vi "Autonomous Independent.vi"() -> ()   [LabVIEW 2015]
doc: "This VI is called when autonomous begins, and will automatically be terminated when autonomous ends. You can carry out timed or sensor driven robot movement independently without needing to return to the caller."
uses:
  <vilib>/Rock Robotics/WPI/Utilities/WPI_GetSetVariantRefNum.vi
  <vilib>/Rock Robotics/Network Tables/NT Read String.vi
  <vilib>/Rock Robotics/Network Tables/NT Write Numeric Array.vi
  <vilib>/Rock Robotics/WPI/RobotDrive/WPI_RobotDriveArcadeDrive_Standard(NoSaturation).vi
  Robot Global Data.vi
panel:
  out "Current Movement, for debugging":T1 {"Y Joystick Value" scale=1.0..-1.0; "X Joystick Value" scale=-1.0..1.0}
  in  "Array of robot movements":T2(array[cluster])=[{"X Joystick Value"=0.39393939393939403, "Y Joystick Value"=0.0, "Delay (sec)"=1.0, "Movement Name"="turn"}, {"X Joystick Value"=-0.3737373737373737, "Y Joystick Value"=0.0, "Delay (sec)"=1.0, "Movement Name"="turn back"}] {"Y Joystick Value" scale=1.0..-1.0; "X Joystick Value" scale=-1.0..1.0}
  # "Be sure to right-click and choose Data Operations>>Make Current Value default if you want to save the array values with the VI"
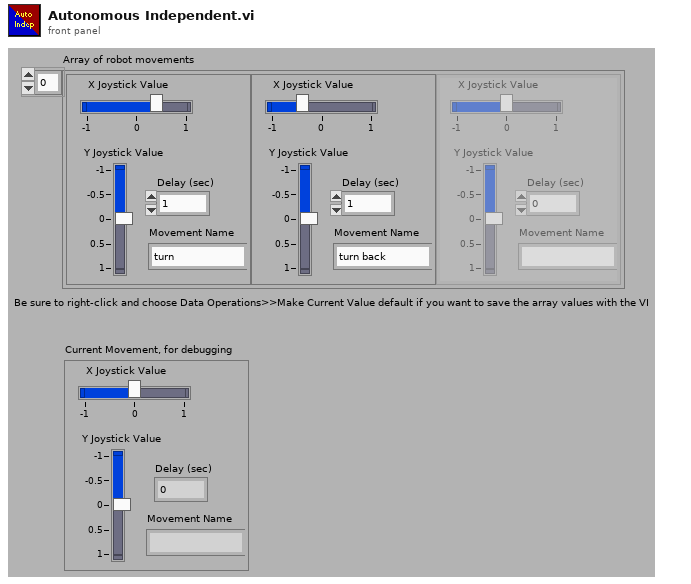
[diagram p1: front panel]
types:
  T1 = cluster{"X Joystick Value":dbl, "Y Joystick Value":dbl, "Delay (sec)":dbl, "Movement Name":string}
  T2 = cluster{"X Joystick Value":dbl, "Y Joystick Value":dbl, "Delay (sec)":dbl, "Movement Name":string}[]
  T3 = typedef "WPI_RobotDriveDevRef.ctl" = cluster{"DevStatus":errorcluster, "Motors[]":T4[], "Square Inputs":bool, "Max Output":dbl}
  T4 = typedef "WPI_MotorControlDeviceRef.ctl" = cluster{"DeviceStatus":errorcluster, "Type":T5, "PWM":cluster{"PWM Channel":T6, "DeadBand":T7}, "CAN":cluster{"Device Number":u8, "Control Mode":T8, "Semaphore":T9, "Max Vout":dbl, "TalonSRX Control Mode":T10}, "Invert":bool}
  T5 = typedef "WPI_MotorControlType.ctl" = enum16{"PWM", "CAN", "CANTalonSRX"}
  T6 = typedef "FPGA_DIOPWMChannel.ctl" = enum8{"PWM 0", "PWM 1", "PWM 2", "PWM 3", "PWM 4", "PWM 5", "PWM 6", "PWM 7", "PWM 8", "PWM 9", "PWM MXP 0", "PWM MXP 1", "PWM MXP 2", "PWM MXP 3", "PWM MXP 4", "PWM MXP 5", "PWM MXP 6", "PWM MXP 7", "PWM MXP 8", "PWM MXP 9", "Invalid"}
  T7 = typedef "WPI_PWMDeadband.ctl" = cluster{"Name":string, "maxPositivePwm":i32, "minPositivePwm":i32, "centerPwm":i32, "maxNegativePwm":i32, "minNegativePwm":i32, "angularRange":u16}
  T8 = typedef "WPI_CANJaguar_ControlMode.ctl" = enum8{"Percent VBus", "Current", "Speed", "Position", "Voltage"}
  T9 = typedef "Semaphore RefNum" = refnum<k1>
  T10 = typedef "WPI_CANTalonSRX_APIControlMode.ctl" = enum8{"Percent VBus", "Speed", "Position", "Slave", "Unchanged / Invalid", "Voltage Compensation", "Current", "Motion Profile"}
  T11 = typedef "WPI_JoystickDevRef.ctl" = cluster{"Device":T12}
  T12 = typedef "WPI_JoystickDeviceEnum.ctl" = enum16{"USB 0", "USB 1", "USB 2", "USB 3", "USB 4", "USB 5"}
  T13 = cluster{"Arm Movement Operation":enum16{"Move to Lower Switch", "Move to Upper Switch", "Move to Sensor Count"}, "Target Sensor Count":i32}
  T14 = cluster{"Drive Operation":enum16{"Turn Robot", "Drive Straight for Time"}, "Turn Angle":dbl, "Drive Time":dbl, "Forward Speed":dbl}
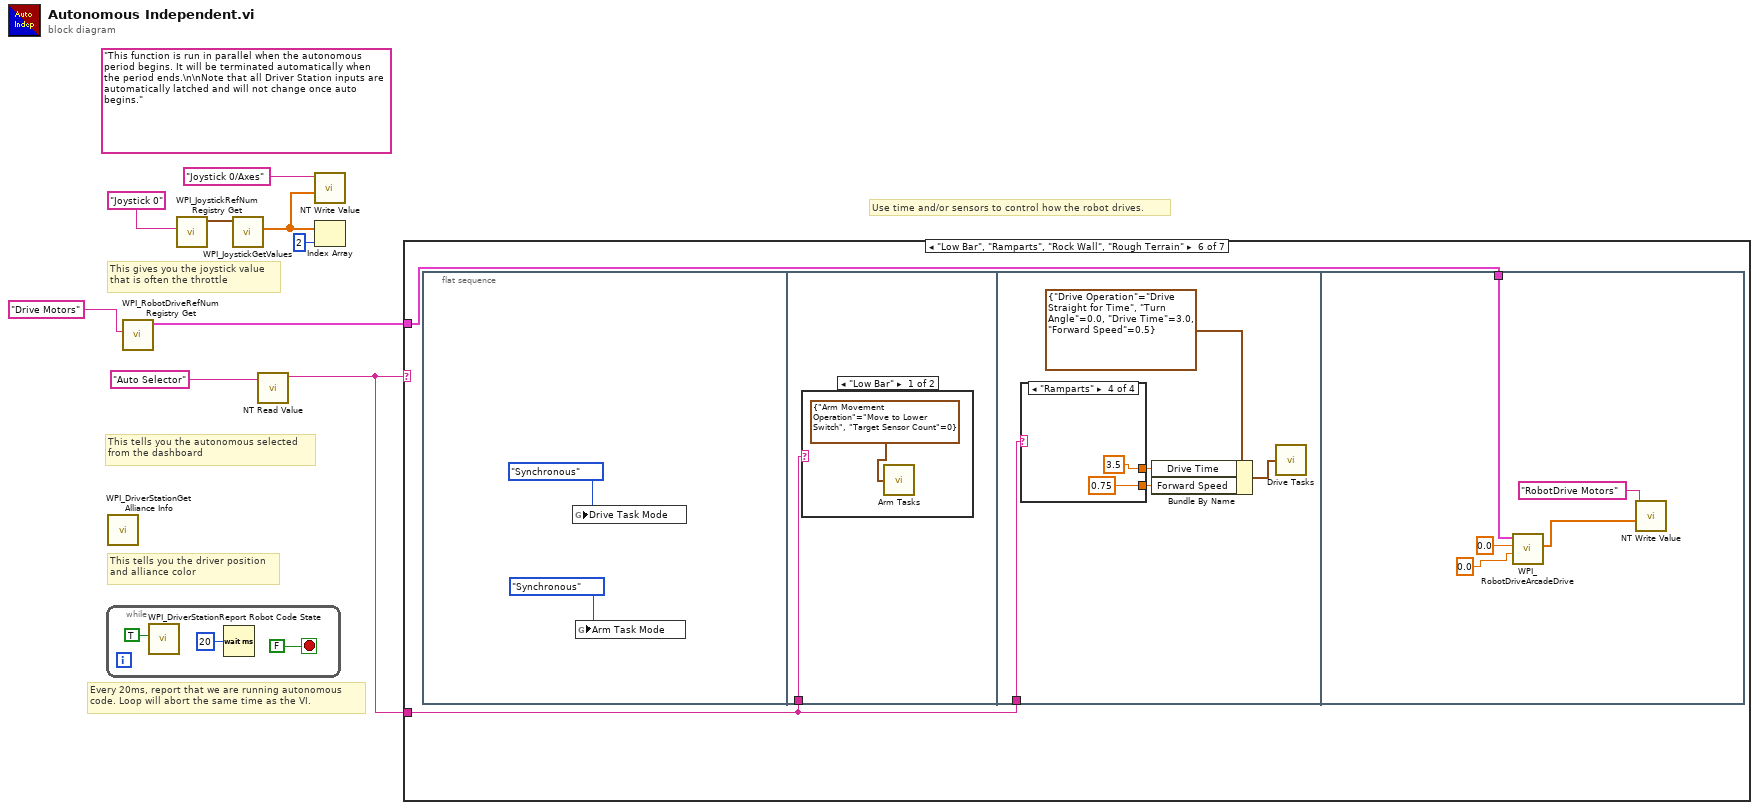
[diagram p0: block diagram]
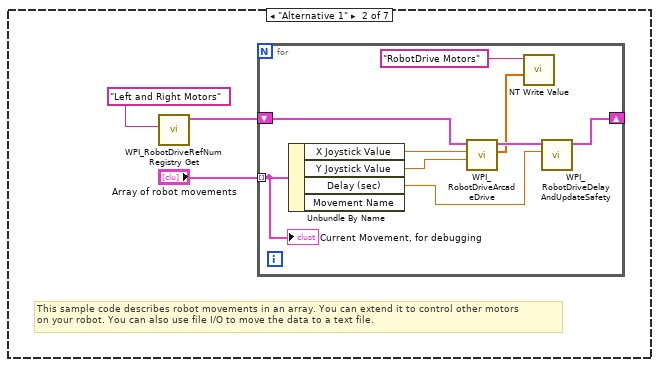
[diagram p3: hidden frame]
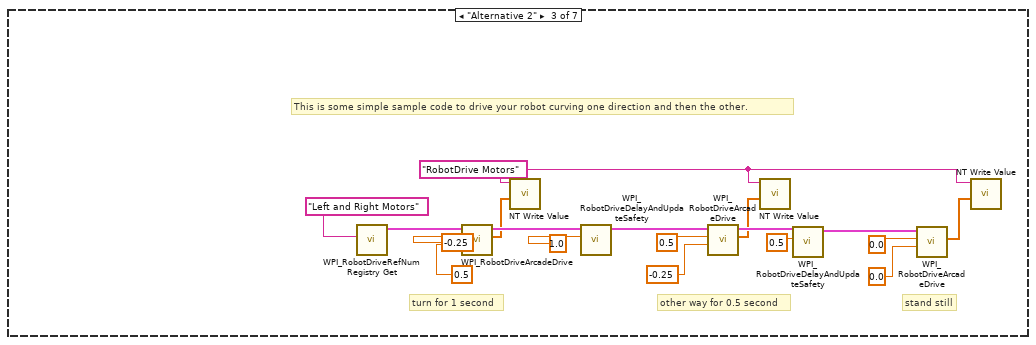
[diagram p4: hidden frame]
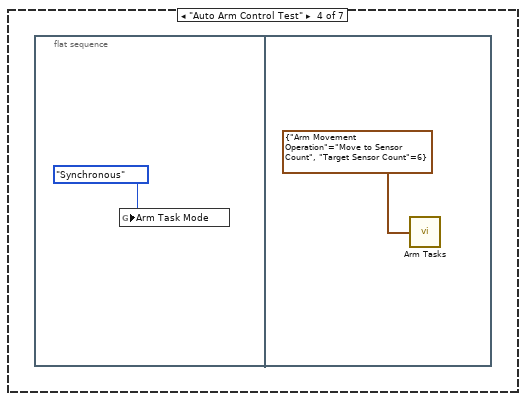
[diagram p5: hidden frame]
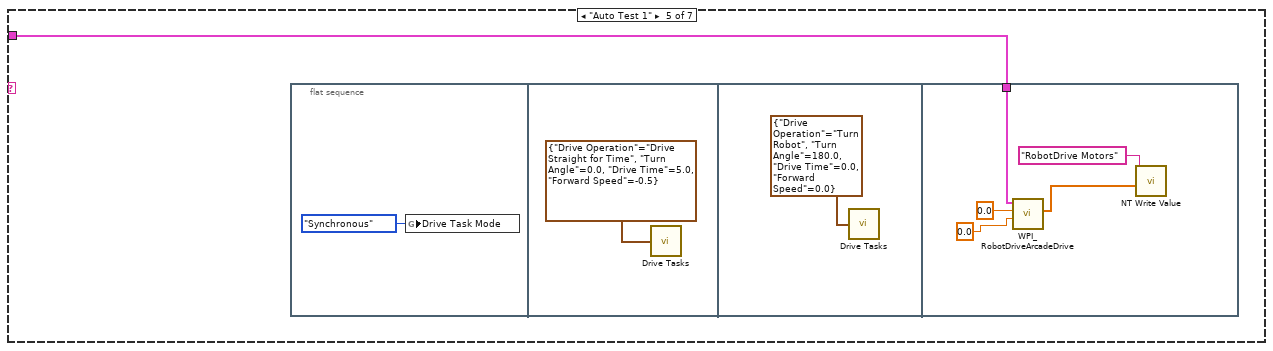
[diagram p6: hidden frame]
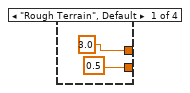
[diagram p8: hidden frame]
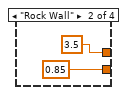
[diagram p9: hidden frame]
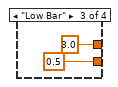
[diagram p10: hidden frame]
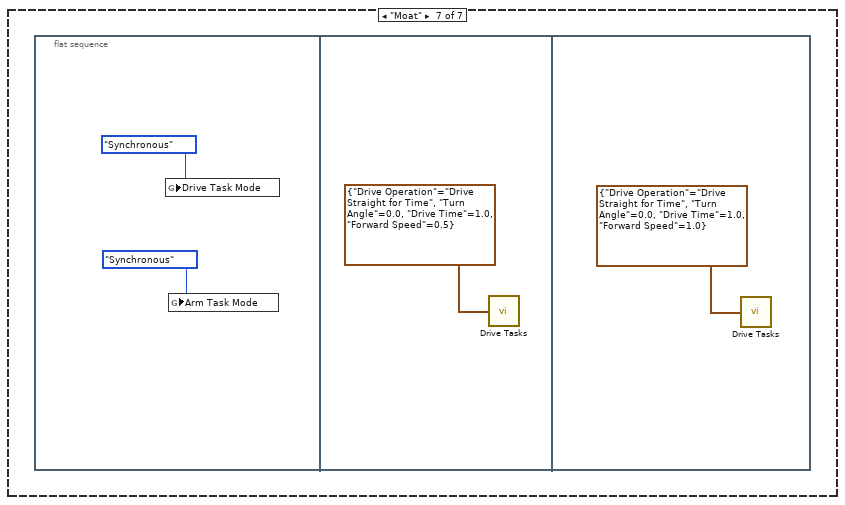
[diagram p11: hidden frame]
diagram:
  (unwired) "This function is run in parallel when the autonomous period begins. It will be terminated automatically when the period ends.\n\nNote that all Driver Station inputs are automatically latched and will not change once auto begins."
  # "This tells you the autonomous selected\nfrom the dashboard"
  # "Every 20ms, report that we are running autonomous\ncode. Loop will abort the same time as the VI."
  # "This gives you the joystick value\nthat is often the throttle"
  # "Use time and/or sensors to control how the robot drives."
  # "This tells you the driver position\nand alliance color"
  n1 = while {
    stop <- FALSE stop-if-true
    n2 = call <vilib>:"WPI_DriverStationReport Robot Code State.vi"("Autonomous"=TRUE) -> ()  [unwired: 10 in, 1 out]
    n3 = Wait (ms)(milliseconds to wait=u32 20) -> ()  [unwired: 1 out]
  }
  n4 = call <vilib>:"WPI_DriverStationGet Alliance Info.vi"() -> ()  [unwired: 12 out]
  n5 = call <vilib>:"WPI_RobotDriveRefNum Registry Get.vi"("refnum name"="Drive Motors") -> ("RobotDriveDevRef"=w2:T3)  [unwired: 9 in, 1 out]
  n6 = call <vilib>:"WPI_JoystickRefNum Registry Get.vi"("refnum name"="Joystick 0") -> ("JoystickDevRef"=w8:T11)  [unwired: 1 in, 9 out]
  n7 = call <vilib>:"WPI_JoystickGetValues.vi"("JoystickDevRef"=w8) -> ("Axes"=w5:dbl[])  [unwired: 6 in, 4 out]
  n8 = call-poly <vilib>:"NT Read Value.vi"("Name"="Auto Selector") -> ("String"=w1:string)  [unwired: 9 in, 1 out]
  n9 = call-poly <vilib>:"NT Write Value.vi"("Numeric Array"=w5, "Name"="Joystick 0/Axes") -> ()  [unwired: 9 in, 1 out]
  n10 = Index Array(array=w5, index=2) -> ()  [unwired: 1 out]
  n11 = case shown="\"Low Bar\", \"Ramparts\", \"Rock Wall\", \"Rough Terrain\"" w1 {
    tunnel: w2 -> [_ _ _ _ w45 w55 _]
    tunnel: w1 -> [_ _ _ _ _ w54 _]
    frame Default {
      # "You can put your main auto here, or you can right-click on the case and make any\nother frame be the default case."
      # "This is the frame that will execute if no selection is made, or if it is not recognized"
    }
    frame "Alternative 1" {
      # "This sample code describes robot movements in an array. You can extend it to control other motors\non your robot. You can also use file I/O to move the data to a text file."
      n12 = call <vilib>:"WPI_RobotDriveRefNum Registry Get.vi"("refnum name"="Left and Right Motors") -> ("RobotDriveDevRef"=w14:T3)  [unwired: 1 in, 9 out]
      n13 = for {
        shift-right: [w22] -> _
        shift-left: w14 -> [w23]
        tunnel: "Array of robot movements" -> [w18] mode=indexing
        n14 = Unbundle By Name(w18) -> ("X Joystick Value"=w21:dbl, "Y Joystick Value"=w20:dbl, "Delay (sec)"=w19:dbl)  [unwired: 1 out]
        n15 = call-poly <vilib>:"WPI_RobotDriveArcadeDrive.vi"("Y axis value"=w20, "X axis value"=w21, "RobotDriveDevRef"=w23) -> ("Motor Values"=w16:dbl[], "RobotDriveDevRef"=w24:T3)  [unwired: 1 in, 6 out]
        n16 = call-poly <vilib>:"NT Write Value.vi"("Numeric Array"=w16, "Name"="RobotDrive Motors") -> ()  [unwired: 9 in, 1 out]
        n17 = call <vilib>:"WPI_RobotDriveDelayAndUpdateSafety.vi"("Delay (s)"=w19, "RobotDriveDevRef"=w24) -> ("RobotDriveDevRef 2"=w22:T3)  [unwired: 8 in, 1 out]
        "Current Movement, for debugging" <- w18
      }
    }
    frame "Alternative 2" {
      w26 = "RobotDrive Motors" ("Name")
      # "This is some simple sample code to drive your robot curving one direction and then the other."
      # "stand still"
      # "other way for 0.5 second"
      # "turn for 1 second"
      n18 = call <vilib>:"WPI_RobotDriveRefNum Registry Get.vi"("refnum name"="Left and Right Motors") -> ("RobotDriveDevRef"=w42:T3)  [unwired: 1 in, 9 out]
      n19 = call-poly <vilib>:"WPI_RobotDriveArcadeDrive.vi"("Y axis value"=0.5 ("X axis value"), "X axis value"=-0.25, "RobotDriveDevRef"=w42) -> ("Motor Values"=w25:dbl[], "RobotDriveDevRef"=w35:T3)  [unwired: 1 in, 6 out]
      n20 = call-poly <vilib>:"NT Write Value.vi"("Numeric Array"=w25, "Name"=w26) -> ()  [unwired: 9 in, 1 out]
      n21 = call <vilib>:"WPI_RobotDriveDelayAndUpdateSafety.vi"("Delay (s)"=1.0, "RobotDriveDevRef"=w35) -> ("RobotDriveDevRef 2"=w36:T3)  [unwired: 8 in, 1 out]
      n22 = call-poly <vilib>:"WPI_RobotDriveArcadeDrive.vi"("Y axis value"=-0.25 ("X axis value"), "X axis value"=0.5, "RobotDriveDevRef"=w36) -> ("Motor Values"=w27:dbl[], "RobotDriveDevRef"=w37:T3)  [unwired: 1 in, 6 out]
      n23 = call-poly <vilib>:"NT Write Value.vi"("Numeric Array"=w27, "Name"=w26) -> ()  [unwired: 9 in, 1 out]
      n24 = call <vilib>:"WPI_RobotDriveDelayAndUpdateSafety.vi"("Delay (s)"=0.5, "RobotDriveDevRef"=w37) -> ("RobotDriveDevRef 2"=w38:T3)  [unwired: 8 in, 1 out]
      n25 = call-poly <vilib>:"WPI_RobotDriveArcadeDrive.vi"("Y axis value"=0.0 ("X axis value"), "X axis value"=0.0, "RobotDriveDevRef"=w38) -> ("Motor Values"=w28:dbl[])  [unwired: 1 in, 7 out]
      n26 = call-poly <vilib>:"NT Write Value.vi"("Numeric Array"=w28, "Name"=w26) -> ()  [unwired: 9 in, 1 out]
    }
    frame "Auto Arm Control Test" {
      n27 = flat-sequence {
        frame #0 {
          n28 = global write "Robot Global Data.vi" "Arm Task Mode"(enum16{"Synchronous", "Asynchronous"}."Synchronous" ("Drive Task Mode")) -> ()
        }
        frame #1 {
          n29 = call "Arm Tasks.vi"("Arm Movement Parameters"=T13 {"Arm Movement Operation"=enum."Move to Sensor Count", "Target Sensor Count"=6}) -> ()  [unwired: 1 in]
        }
      }
    }
    frame "Auto Test 1" {
      n30 = flat-sequence {
        tunnel: w45 -> [w53]
        frame #0 {
          n31 = global write "Robot Global Data.vi" "Drive Task Mode"(enum16{"Synchronous", "Asynchronous"}."Synchronous" ("Drive Task Mode")) -> ()
        }
        frame #1 {
          n32 = call "Drive Tasks.vi"("Drive Parameters"=T14 {"Drive Operation"=enum."Drive Straight for Time", "Turn Angle"=0.0, "Drive Time"=5.0, "Forward Speed"=-0.5}) -> ()  [unwired: 1 in]
        }
        frame #2 {
          n33 = call "Drive Tasks.vi"("Drive Parameters"=T14 {"Drive Operation"=enum."Turn Robot", "Turn Angle"=180.0, "Drive Time"=0.0, "Forward Speed"=0.0}) -> ()  [unwired: 1 in]
        }
        frame #3 {
          n34 = call-poly <vilib>:"WPI_RobotDriveArcadeDrive.vi"("Y axis value"=0.0, "X axis value"=0.0, "RobotDriveDevRef"=w53) -> ("Motor Values"=w49:dbl[])  [unwired: 6 in, 2 out]
          n35 = call-poly <vilib>:"NT Write Value.vi"("Numeric Array"=w49, "Name"="RobotDrive Motors") -> ()  [unwired: 9 in, 1 out]
        }
      }
    }
    frame "Low Bar", "Ramparts", "Rock Wall", "Rough Terrain" {
      n36 = flat-sequence {
        tunnel: w54 -> [w58]
        tunnel: w54 -> [w62]
        tunnel: w55 -> [w73]
        frame #0 {
          n37 = global write "Robot Global Data.vi" "Drive Task Mode"(enum16{"Synchronous", "Asynchronous"}."Synchronous" ("Drive Task Mode")) -> ()
          n38 = global write "Robot Global Data.vi" "Arm Task Mode"(enum16{"Synchronous", "Asynchronous"}."Synchronous" ("Drive Task Mode")) -> ()
        }
        frame #1 {
          n39 = case shown="\"Low Bar\"" w58 {
            frame "Low Bar" {
              n40 = call "Arm Tasks.vi"("Arm Movement Parameters"=T13 {"Arm Movement Operation"=enum."Move to Lower Switch", "Target Sensor Count"=0}) -> ()  [unwired: 1 in]
            }
            frame Default {
            }
          }
        }
        frame #2 {
          n41 = case shown="\"Ramparts\"" w62 {
            tunnel: [3.0 ("Drive Time") 3.5 ("Drive Time") 3.0 ("Drive Time") 3.5 ("Drive Time")] -> w61
            tunnel: [0.5 0.85 0.5 0.75] -> w60
            frame "Rough Terrain", Default {
            }
            frame "Rock Wall" {
            }
            frame "Low Bar" {
            }
            frame "Ramparts" {
            }
          }
          n42 = Bundle By Name(cluster=T14 {"Drive Operation"=enum."Drive Straight for Time", "Turn Angle"=0.0, "Drive Time"=3.0, "Forward Speed"=0.5} ("Drive Parameters"), "Drive Time"=w61, "Forward Speed"=w60) -> (w63:T14)
          n43 = call "Drive Tasks.vi"("Drive Parameters"=w63) -> ()  [unwired: 1 in]
        }
        frame #3 {
          n44 = call-poly <vilib>:"WPI_RobotDriveArcadeDrive.vi"("Y axis value"=0.0, "X axis value"=0.0, "RobotDriveDevRef"=w73) -> ("Motor Values"=w74:dbl[])  [unwired: 6 in, 2 out]
          n45 = call-poly <vilib>:"NT Write Value.vi"("Numeric Array"=w74, "Name"="RobotDrive Motors") -> ()  [unwired: 9 in, 1 out]
        }
      }
    }
    frame "Moat" {
      n46 = flat-sequence {
        frame #0 {
          n47 = global write "Robot Global Data.vi" "Drive Task Mode"(enum16{"Synchronous", "Asynchronous"}."Synchronous" ("Drive Task Mode")) -> ()
          n48 = global write "Robot Global Data.vi" "Arm Task Mode"(enum16{"Synchronous", "Asynchronous"}."Synchronous" ("Drive Task Mode")) -> ()
        }
        frame #1 {
          n49 = call "Drive Tasks.vi"("Drive Parameters"=T14 {"Drive Operation"=enum."Drive Straight for Time", "Turn Angle"=0.0, "Drive Time"=1.0, "Forward Speed"=0.5}) -> ()  [unwired: 1 in]
        }
        frame #2 {
          n50 = call "Drive Tasks.vi"("Drive Parameters"=T14 {"Drive Operation"=enum."Drive Straight for Time", "Turn Angle"=0.0, "Drive Time"=1.0, "Forward Speed"=1.0}) -> ()  [unwired: 1 in]
        }
      }
    }
  }
